vi "UnscentedKalmanFilter_Correct_OnlyUY.vi"(4 "H_ExtraData":variant, 6 "H_Func":T1, 9 "Y":T2, 10 "U":T2, 11 "in UnscentedKalmanFiilter":T3) -> (0 "Error":bool, 3 "out UnscentedKalmanFiilter":T3)   [LabVIEW 2019, in "Trajectory_Library.lvlib"]
doc: "Correct the state estimate x-hat using the measurements in y.\n \nInputs:\n - inUnscentedKalmanFilter -- filter data cluster\n - u -- Same control input used in the predict step.\n - y -- Measurement vector.\n - H_Func -- A vector-valued function of x and u that returns the measurement vector.\n - H_ExtraData -- Variant containing extra data used by the H function. The contents of the variant are specific to the H function.\n\n\nOutputs:\n - outUnscentedKalmanFilter -- updated filter data cluster\n - Error -- If TRUE, an error occured."
uses:
  Trajectory_Library.lvlib
  TypeDef/UNSCENTED_KALMAN_FILTER.ctl
  <vilib>/Analysis/Matrix/Datatypes/RealMatrix.ctl
  TypeDef/MERWE_SCALED_SIGMA_PTS.ctl
  TypeDef/CALLBACK_FUNC_TYPE.ctl
  <vilib>/Analysis/Matrix/NI_Matrix.lvlib
panel:
  # "<Inputs, 1>"
  # "<Outputs, 1>"
  # "State Estimate <Statess,1>"
  # "<States, States>"
  # "<States, ?>"
  # "<Statess,  States>"
  # "<Outputs, Outputs>"
  # "<?, 1>"
  # "<?, 1>"
  # "State Estimate <Statess,1>"
  # "<States, States>"
  # "<States, ?>"
  # "<Statess,  States>"
  # "<Outputs, Outputs>"
  # "<?, 1>"
  # "<?, 1>"
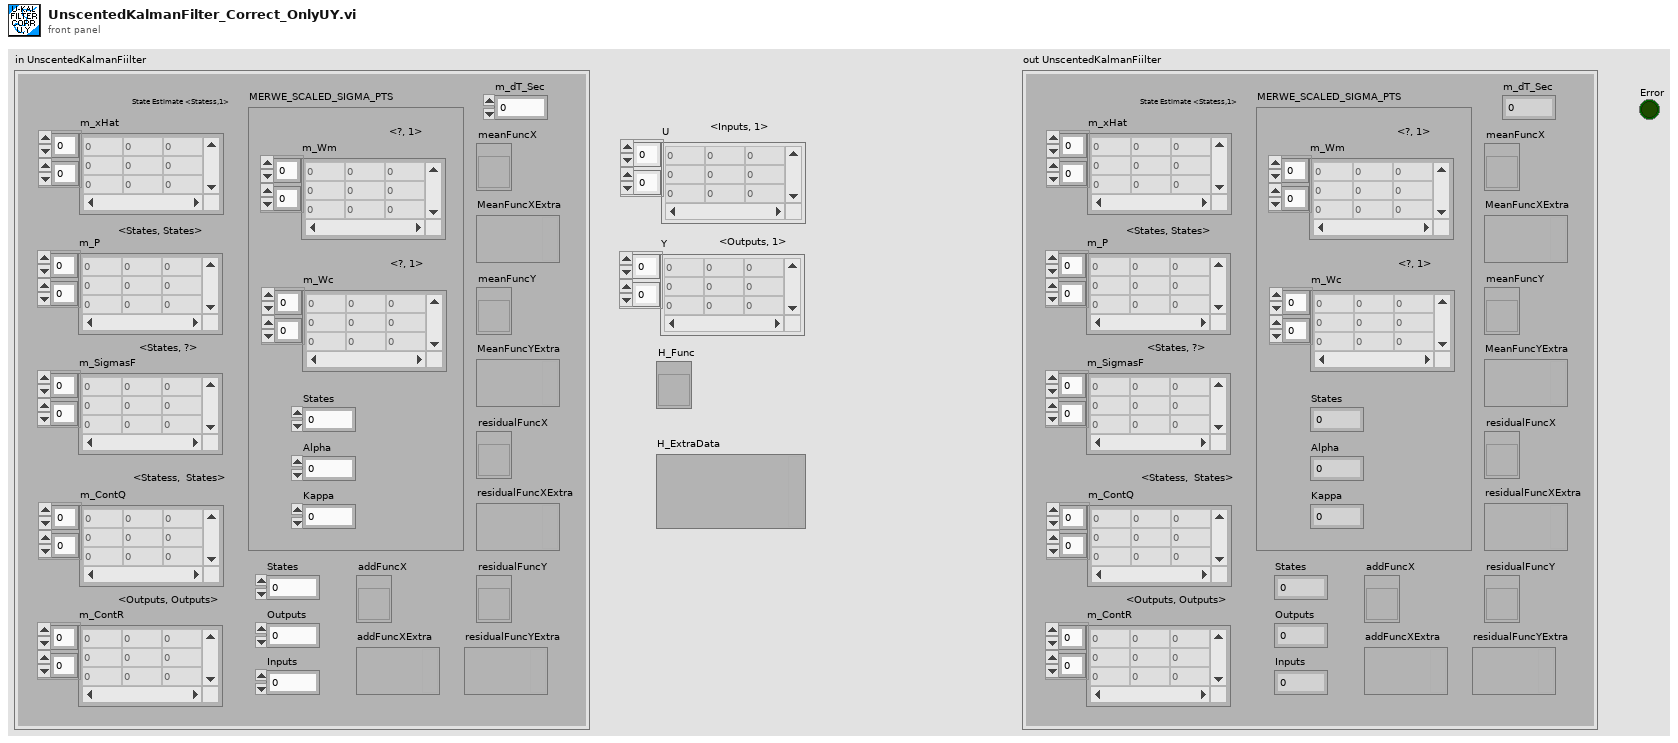
[diagram p1: front panel]
types:
  T1 = typedef "Trajectory_Library.lvlib/CALLBACK_FUNC_TYPE.ctl" = refnum<vi>
  T2 = typedef "NI_Matrix.lvlib/RealMatrix.ctl" = dbl[][]
  T3 = typedef "Trajectory_Library.lvlib/UNSCENTED_KALMAN_FILTER.ctl" = cluster{"m_P":T2, "m_xHat":T2, "States":i32, "Outputs":i32, "m_ContR":T2, "m_ContQ":T2, "m_SigmasF":T2, "m_dT_Sec":dbl, "MERWE_SCALED_SIGMA_PTS":T4, "meanFuncX":T1, "meanFuncY":T1, "residualFuncX":T1, "residualFuncY":T1, "addFuncX":T1, "addFuncXExtra":variant, "residualFuncYExtra":variant, "residualFuncXExtra":variant, "MeanFuncYExtra":variant, "MeanFuncXExtra":variant, "Inputs":i32}
  T4 = typedef "Trajectory_Library.lvlib/MERWE_SCALED_SIGMA_PTS.ctl" = cluster{"m_Wm":T2, "States":i32, "Alpha":dbl, "m_Wc":T2, "Kappa":i32}
  T5 = typedef "Trajectory_Library.lvlib/UNSCENTED_KALMAN_CORRECT_FUNC_GROUP.ctl" = cluster{"H_Func":T1, "meanFuncY":T1, "residualFuncY":T1, "residualFuncX":T1, "addFuncX":T1, "H_FuncExtra":variant, "MeanFuncYExtra":variant, "residualFuncYExtra":variant, "residualFuncXExtra":variant, "addFuncXExtra":variant}
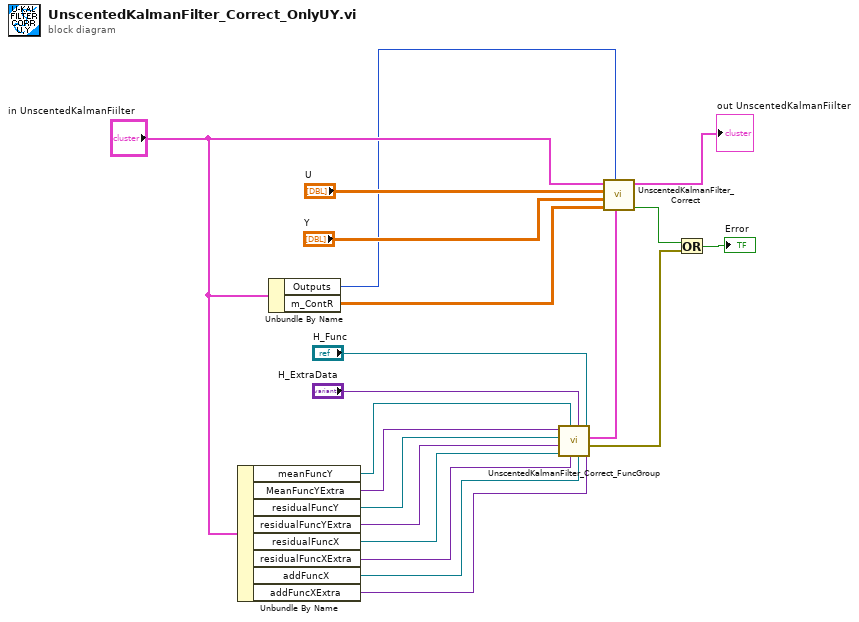
[diagram p0: block diagram]
diagram:
  n1 = Unbundle By Name("in UnscentedKalmanFiilter") -> ("meanFuncY"=w14:T1, "MeanFuncYExtra"=w13:variant, "residualFuncY"=w12:T1, "residualFuncYExtra"=w11:variant, "residualFuncX"=w10:T1, "residualFuncXExtra"=w9:variant, "addFuncX"=w8:T1, "addFuncXExtra"=w7:variant)
  n2 = Unbundle By Name("in UnscentedKalmanFiilter") -> ("Outputs"=w5:i32, "m_ContR"=w4:T2)
  n3 = call "UnscentedKalmanFilter_Correct_FuncGroup.vi"("addFuncXExtra"=w7, "H_Func"="H_Func", "AddFuncX"=w8, "H_FuncExtra"="H_ExtraData", "residualFuncXExtra"=w9, "MeanFuncY"=w14, "ResidualFuncX"=w10, "residualFuncYExtra"=w11, "ResidualFuncY"=w12, "MeanFuncYExtra"=w13) -> ("Error"=w1:errorcluster, "UNSCENTED_KALMAN_CORRECT_FUNC_GROUP"=w17:T5)
  n4 = call "UnscentedKalmanFilter_Correct.vi"("UNSCENTED_KALMAN_CORRECT_FUNC_GROUP"=w17, "Rows"=w5, "R"=w4, "Y"="Y", "U"="U", "in UnscentedKalmanFiilter"="in UnscentedKalmanFiilter") -> ("Error"=w2:bool, "out UnscentedKalmanFiilter"=→"out UnscentedKalmanFiilter":T3)  [unwired: 4 in]
  n5 = Or(x=w2, y=w1) -> (x .or. y?=→"Error":bool)
